vi "UNIT_Ex.vi"(10 "In":string) -> (2 "Out":string)   [LabVIEW 2017]
panel:
  in  "Txt 1":string="deg"
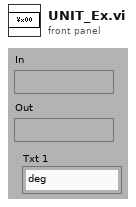
[diagram p1: front panel]
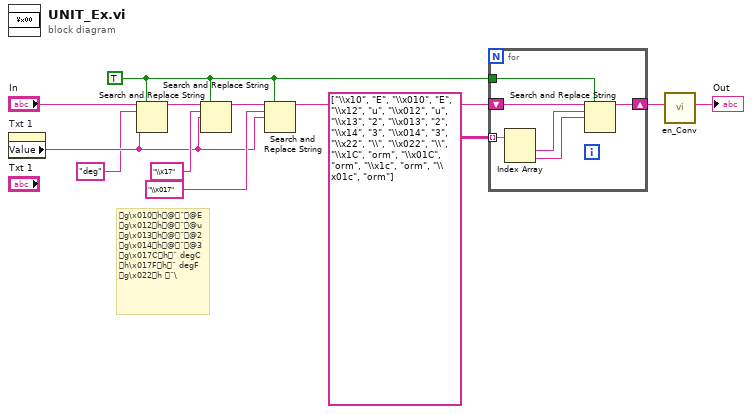
[diagram p0: block diagram]
diagram:
  w3 = TRUE ("replace all? (F)")
  # "g\\x010h@¨@E\ng\\x012h@¨@u\ng\\x013h@¨@2\ng\\x014h@¨@3\ng\\x017Ch¨ degC\nh\\x017Fh¨ degF\ng\\x022h ¨\\"
  n1 = property on="Txt 1" class="Str"() -> ("Value"=w5:string)  [unwired: 2 in, 2 out]
  n2 = Search and Replace String(replace all?=w3, input string="In", search string="deg" ("regular expression"), replace string=w5) -> (result string=w7:string)  [unwired: 1 in, 6 out]
  n3 = Search and Replace String(replace all?=w3, input string=w7, search string="\\x17" ("regular expression"), replace string=w5) -> (result string=w11:string)  [unwired: 1 in, 6 out]
  n4 = Search and Replace String(replace all?=w3, input string=w11, search string="\\x017" ("regular expression"), replace string=w5) -> (result string=w10:string)  [unwired: 1 in, 6 out]
  n5 = for {
    tunnel: w3 -> [w17]
    tunnel: string[][] [["\\x10", "E"], ["\\x010", "E"], ["\\x12", "u"], ["\\x012", "u"], ["\\x13", "2"], ["\\x013", "2"], ["\\x14", "3"], ["\\x014", "3"], ["\\x22", "\\"], ["\\x022", "\\"], ["\\x1C", "orm"], ["\\x01C", "orm"], ["\\x1c", "orm"], ["\\x01c", "orm"]] -> [w15] mode=indexing
    shift-right: [w16] -> w2
    shift-left: w10 -> [w18]
    n6 = Index Array(array=w15) -> (element #1=w14:string, element #2=w13:string)  [unwired: 2 in]
    n7 = Search and Replace String(replace all?=w17, input string=w18, search string=w14, replace string=w13) -> (result string=w16:string)  [unwired: 1 in, 6 out]
  }
  n8 = call "en_Conv.vi"("In"=w2) -> ("Out"=→"Out":string)  [unwired: 1 in, 9 out]
